vi "start acquisition.vi"(8 "error in (no error)":errorcluster, 9 "Image Type":T1=1 items=["Grayscale (U8)", "Grayscale (I16)", "Grayscale (SGL)", "Complex (CSG)", "RGB (U32)", "HSL (U32)", "RGB (U64)", "Grayscale (U16)"], 10 "Camera Name":T2, 11 "IMAQdx Cam in":refnum<class "IMAQdx Cam.lvclass">) -> (0 "error out":errorcluster, 2 "Event Registration Refnum":refnum<event-registration>, 3 "IMAQdx Cam out":refnum<class "IMAQdx Cam.lvclass">)   [LabVIEW 2009, in "IMAQdx Cam.lvclass"]
uses:
  IMAQdx Cam.lvclass
  <vilib>/userDefined/High Color/IMAQdx.ctl
  <vilib>/vision/driver/IMAQdx.llb/IMAQdx Acquisition Mode.ctl
  <vilib>/vision/driver/IMAQdx.llb/IMAQdx Camera Control Mode.ctl
  IMAQdx Cam.lvclass/IMAQdx Cam.ctl
  <vilib>/vision/driver/NI_Vision_Acquisition_Software.lvlib
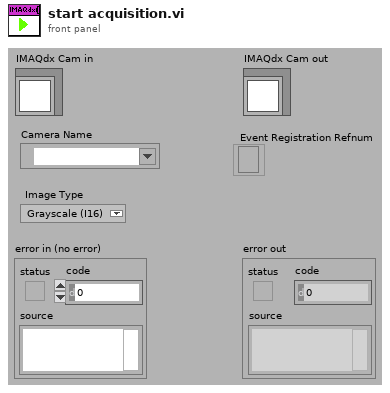
[diagram p1: front panel]
types:
  T1 = typedef "Image Type" = u32
  T2 = typedef "IMAQdx.ctl" = refnum<k21>
  T3 = typedef "NI_Vision_Acquisition_Software.lvlib/IMAQdx Acquisition Mode.ctl" = enum32{"One Shot", "Continuous"}
  T4 = typedef "NI_Vision_Acquisition_Software.lvlib/IMAQdx Camera Control Mode.ctl" = enum32{"Controller", "Listener"}
  T5 = typedef "IMAQ Image.ctl" = refnum<image>
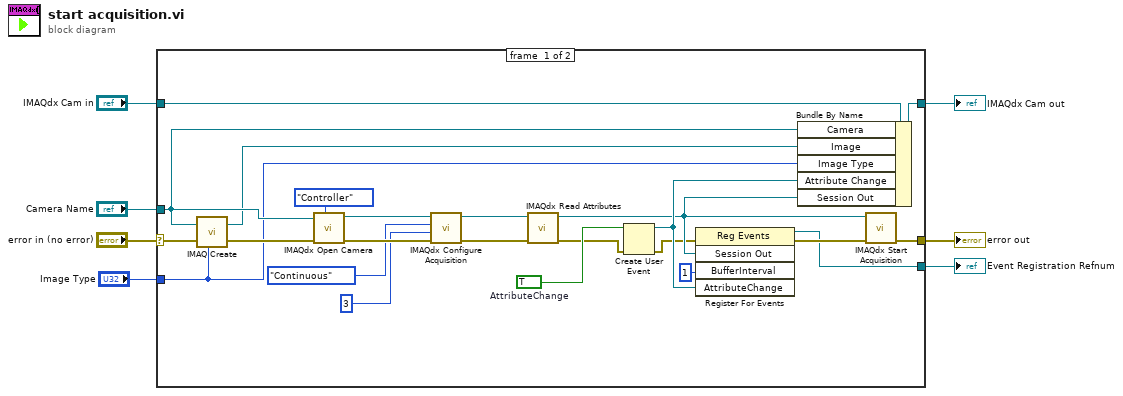
[diagram p0: block diagram]
diagram:
  n1 = case shown="No Error" "error in (no error)" {
    selector: "error in (no error)" -> [w20 w32]
    tunnel: [w24 w32] -> w6
    tunnel: [w22 w31] -> w4
    tunnel: "IMAQdx Cam in" -> [w23 w31]
    tunnel: "Camera Name" -> [w21 _]
    tunnel: [w16 _] -> w1
    tunnel: "Image Type" -> [w13 _]
    frame #0 {
      w15 = TRUE  # AttributeChange
      n2 = call "IMAQ Create"("Image Name"=w21, "Image Type"=w13, "error in (no error)"=w20) -> ("New Image"=w18:T5, "error out"=w19:errorcluster)  [unwired: 1 in, 1 out]
      n3 = call <vilib>:"IMAQdx Open Camera.vi"("Camera Control Mode"=IMAQdx_Camera_Control_Mode."Controller", "error in"=w19, "Session In"=w21) -> ("error out"=w28:errorcluster, "Session Out"=w29:T2)  [unwired: 7 out]
      n4 = call <vilib>:"IMAQdx Configure Acquisition.vi"("error in"=w28, "Number of Buffers"=u32 3, "Continuous?"=IMAQdx_Acquisition_Mode."Continuous", "Session In"=w29) -> ("error out"=w10:errorcluster, "Session Out"=w12:T2)  [unwired: 6 out]
      n5 = call <vilib>:"IMAQdx Read Attributes.vi"("error in"=w10, "Session In"=w12) -> ("error out"=w9:errorcluster, "Session Out"=w11:T2)  [unwired: 8 in]
      n6 = Create User Event(user event datatype=w15, error in=w9) -> (user event=w14:refnum<user-event>, error out=w8:errorcluster)
      n7 = register-events(error in=w8, w11, u32 1 ("BufferInterval"), w14) -> (reference out=w16:refnum<event-registration>, error out=w25:errorcluster)  [unwired: 1 in]
      n8 = Bundle By Name(cluster=w23, "Camera"=w21, "Image"=w18, "Image Type"=w13, "Attribute Change"=w14, "Session Out"=w11) -> (w22:refnum<class "IMAQdx Cam.lvclass">)
      n9 = call <vilib>:"IMAQdx Start Acquisition.vi"("error in"=w25, "Session In"=w11) -> ("error out"=w24:errorcluster)  [unwired: 9 out]
    }
    frame #1 {
    }
  }
  "error out" <- w6
  "IMAQdx Cam out" <- w4
  "Event Registration Refnum" <- w1
